vi "Construct_Optimal_Subtrack_(111)-1.vi"(6 "[IN] Indexes for Jumps":i32[](array[numeric]), 8 "error IN":errorcluster, 9 "[IN] Index of recon\nstructed tracks":i32, 10 "[IN] Clusters for Re\nconstructed Tracks":T1, 11 "[IN] Still connected\ntracks in group":T2) -> (0 "error OUT":errorcluster, 1 "[OUT] Decrease status of connected\nwith 111 points (it's bad point)":bool, 2 "[OUT] Clusters for Re\nconstructed Tracks":T1)   [LabVIEW 2013]
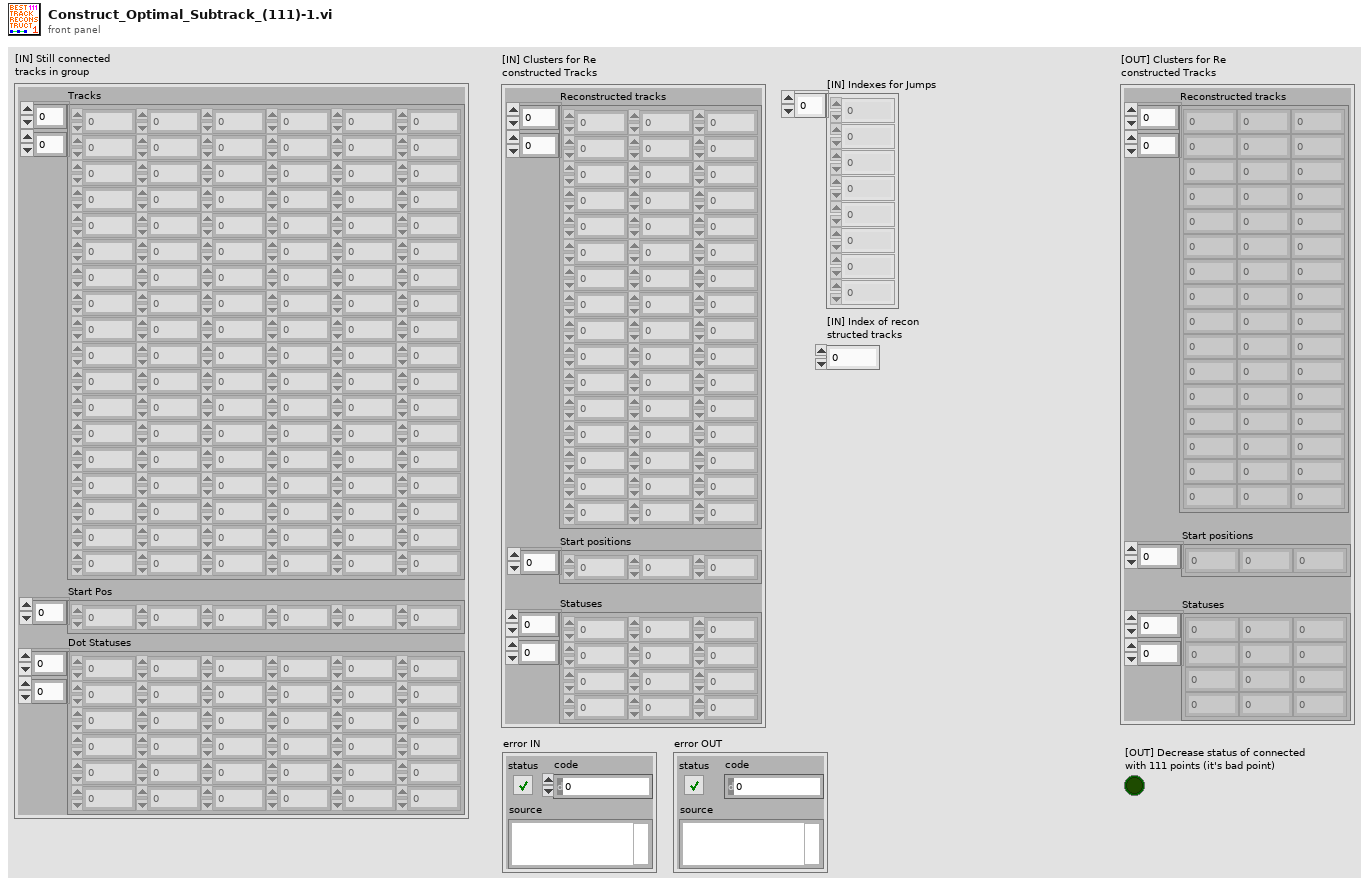
[diagram p1: front panel]
types:
  T1 = cluster{"Reconstructed tracks":dbl[][], "Start positions":i32[], "Statuses":i16[][]}
  T2 = cluster{"Tracks":dbl[][], "Start Pos":i32[], "Dot Statuses":i16[][]}
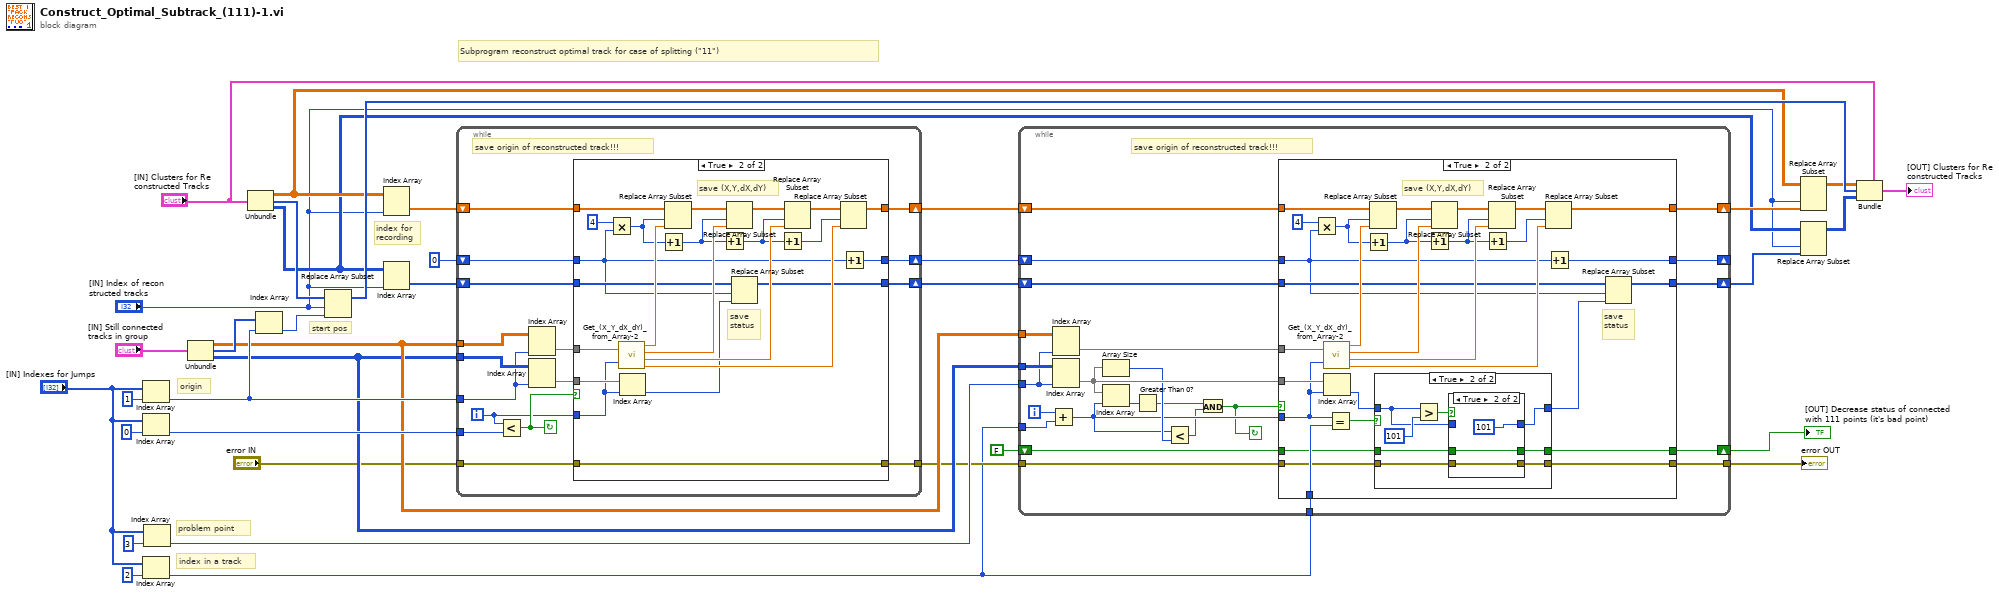
[diagram p0: block diagram]
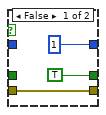
[diagram p4: hidden frame]
diagram:
  # "index in a track"
  # "problem point"
  # "origin"
  # "Subprogram reconstruct optimal track for case of splitting (\"11\")"
  # "index for\nrecording"
  # "start pos"
  n1 = Index Array(array="[IN] Indexes for Jumps", index=1) -> (element=w27:i32)
  n2 = Index Array(array="[IN] Indexes for Jumps", index=0) -> (element=w30:i32)
  n3 = Index Array(array="[IN] Indexes for Jumps", index=2) -> (element=w3:i32)
  n4 = Index Array(array="[IN] Indexes for Jumps", index=3) -> (element=w17:i32)
  n5 = Unbundle("[IN] Still connected\ntracks in group") -> ("Tracks"=w19:dbl[][], "Start Pos"=w28:i32[], "Dot Statuses"=w18:i16[][])
  n6 = Unbundle("[IN] Clusters for Re\nconstructed Tracks") -> ("Reconstructed tracks"=w14:dbl[][], "Start positions"=w29:i32[], "Statuses"=w11:i16[][])
  n7 = Index Array(array=w28, index=w27) -> (element=w26:i32)
  n8 = Replace Array Subset(array=w29, new element=w26, index="[IN] Index of recon\nstructed tracks") -> (w15:i32[])
  n9 = Index Array(array=w14, index (col)="[IN] Index of recon\nstructed tracks") -> (element=w25:dbl[])  [unwired: 1 in]
  n10 = Index Array(array=w11, index (col)="[IN] Index of recon\nstructed tracks") -> (element=w24:i16[])  [unwired: 1 in]
  n11 = while {
    tunnel: w30 -> [w49]
    tunnel: w19 -> [w52]
    tunnel: w18 -> [w51]
    tunnel: w27 -> [w50]
    shift-right: [w41] -> w22
    shift-left: w25 -> [w47]
    shift-right: [w39] -> w20
    shift-left: w24 -> [w43]
    shift-right: [w40] -> w21
    shift-left: 0 -> [w42]
    tunnel: "error IN" -> [w38]
    tunnel: [w37] -> w5
    i -> [w44]
    stop <- w48 continue-if-true
    # "save origin of reconstructed track!!!"
    n12 = Less?(x=w44, y=w49) -> (x < y?=w48:bool)
    n13 = Index Array(array=w52, index (col)=w50) -> (element=w46:dbl[])  [unwired: 1 in]
    n14 = Index Array(array=w51, index (col)=w50) -> (element=w45:i16[])  [unwired: 1 in]
    n15 = case shown="True" w48 {
      tunnel: w47 -> [w56 w77]
      tunnel: w46 -> [_ w79]
      tunnel: w45 -> [_ w78]
      tunnel: w44 -> [_ w62]
      tunnel: w43 -> [w54 w64]
      tunnel: [w54 w61] -> w39
      tunnel: [w56 w60] -> w41
      tunnel: w42 -> [w55 w59]
      tunnel: [w55 w58] -> w40
      tunnel: w38 -> [w53 w57]
      tunnel: [w53 w57] -> w37
      frame False {
      }
      frame True {
        # "save (X,Y,dX,dY)"
        # "save\nstatus"
        n16 = Multiply(x=4, y=w59) -> (x*y=w73:i32)
        n17 = call "Get_(X_Y_dX_dY)_from_Array-2.vi"("(X,Y,dX,dY)"=w79, "Index of Displacement"=w62) -> ("X"=w75:dbl, "Y"=w72:dbl, "dX"=w69:dbl, "dY"=w65:dbl)
        n18 = Index Array(array=w78, index=w62) -> (element=w63:i16)
        n19 = Increment(x=w73) -> (x+1=w70:i32)
        n20 = Replace Array Subset(array=w77, new element=w75, index=w73) -> (w74:dbl[])
        n21 = Increment(x=w70) -> (x+1=w68:i32)
        n22 = Replace Array Subset(array=w74, new element=w72, index=w70) -> (w71:dbl[])
        n23 = Replace Array Subset(array=w64, new element=w63, index=w59) -> (w61:i16[])
        n24 = Increment(x=w68) -> (x+1=w67:i32)
        n25 = Replace Array Subset(array=w71, new element=w69, index=w68) -> (w66:dbl[])
        n26 = Replace Array Subset(array=w66, new element=w65, index=w67) -> (w60:dbl[])
        n27 = Increment(x=w59) -> (x+1=w58:i32)
      }
    }
  }
  n28 = while {
    tunnel: w19 -> [w103]
    tunnel: w18 -> [w102]
    tunnel: w17 -> [w101]
    shift-right: [w96] -> w13
    shift-left: w22 -> [w100]
    shift-right: [w94] -> w10
    shift-left: w20 -> [w98]
    shift-right: [w95] -> _
    shift-left: w21 -> [w97]
    tunnel: w3 -> [w92]
    tunnel: w5 -> [w84]
    tunnel: [w83] -> w4
    tunnel: w3 -> [w82]
    shift-right: [w80] -> w1
    shift-left: FALSE -> [w81]
    i -> [w93]
    stop <- w85 continue-if-true
    # "save origin of reconstructed track!!!"
    n29 = Add(x=w93, y=w92) -> (x+y=w88:i32)
    n30 = Index Array(array=w103, index (col)=w101) -> (element=w99:dbl[])  [unwired: 1 in]
    n31 = Index Array(array=w102, index (col)=w101) -> (element=w91:i16[])  [unwired: 1 in]
    n32 = Array Size(array=w91) -> (size(s)=w89:i32)
    n33 = Index Array(array=w91, index=w88) -> (element=w90:i16)
    n34 = Greater Than 0?(x=w90) -> (x > 0?=w87:bool)
    n35 = Less?(x=w88, y=w89) -> (x < y?=w86:bool)
    n36 = And(x=w87, y=w86) -> (x .and. y?=w85:bool)
    n37 = case shown="True" w85 {
      tunnel: w100 -> [w108 w135]
      tunnel: w99 -> [_ w137]
      tunnel: w91 -> [_ w136]
      tunnel: w88 -> [_ w117]
      tunnel: w98 -> [w106 w122]
      tunnel: [w106 w121] -> w94
      tunnel: [w108 w120] -> w96
      tunnel: w97 -> [w107 w119]
      tunnel: [w107 w118] -> w95
      tunnel: w84 -> [w105 w113]
      tunnel: [w105 w112] -> w83
      tunnel: w82 -> [_ w116]
      tunnel: w81 -> [w104 w110]
      tunnel: [w104 w109] -> w80
      frame False {
      }
      frame True {
        # "save (X,Y,dX,dY)"
        # "save\nstatus"
        n38 = Multiply(x=4, y=w119) -> (x*y=w131:i32)
        n39 = call "Get_(X_Y_dX_dY)_from_Array-2.vi"("(X,Y,dX,dY)"=w137, "Index of Displacement"=w117) -> ("X"=w133:dbl, "Y"=w130:dbl, "dX"=w127:dbl, "dY"=w123:dbl)
        n40 = Index Array(array=w136, index=w117) -> (element=w114:i16)
        n41 = Equal?(x=w117, y=w116) -> (x = y?=w115:bool)
        n42 = Increment(x=w131) -> (x+1=w128:i32)
        n43 = Replace Array Subset(array=w135, new element=w133, index=w131) -> (w132:dbl[])
        n44 = case shown="True" w115 {
          tunnel: w114 -> [w140 w145]
          tunnel: w113 -> [w139 w146]
          tunnel: [w140 w144] -> w111
          tunnel: [w139 w143] -> w112
          tunnel: w110 -> [w138 w142]
          tunnel: [w138 w141] -> w109
          frame False {
          }
          frame True {
            n45 = Greater?(x=w145, y=i16 101) -> (0:w147:bool)
            n46 = case shown="True" w147 {
              tunnel: w146 -> [w151 w153]
              tunnel: w145 -> [_ _]
              tunnel: [i16 1 ("y") i16 101 ("y")] -> w144
              tunnel: [w151 w153] -> w143
              tunnel: w142 -> [_ w152]
              tunnel: [TRUE w152] -> w141
              frame False {
              }
              frame True {
              }
            }
          }
        }
        n47 = Increment(x=w128) -> (x+1=w126:i32)
        n48 = Replace Array Subset(array=w132, new element=w130, index=w128) -> (w129:dbl[])
        n49 = Increment(x=w126) -> (x+1=w125:i32)
        n50 = Replace Array Subset(array=w129, new element=w127, index=w126) -> (w124:dbl[])
        n51 = Replace Array Subset(array=w124, new element=w123, index=w125) -> (w120:dbl[])
        n52 = Increment(x=w119) -> (x+1=w118:i32)
        n53 = Replace Array Subset(array=w122, new element=w111, index=w119) -> (w121:i16[])
      }
    }
  }
  "error OUT" <- w4
  "[OUT] Decrease status of connected\nwith 111 points (it's bad point)" <- w1
  n54 = Replace Array Subset(array=w14, new element=w13, index (col)="[IN] Index of recon\nstructed tracks") -> (w12:dbl[][])  [unwired: 1 in]
  n55 = Replace Array Subset(array=w11, new element=w10, index (col)="[IN] Index of recon\nstructed tracks") -> (w8:i16[][])  [unwired: 1 in]
  n56 = Bundle(cluster="[IN] Clusters for Re\nconstructed Tracks", "Reconstructed tracks"=w12, "Start positions"=w15, "Statuses"=w8) -> (→"[OUT] Clusters for Re\nconstructed Tracks":T1)
